vi "PXI-Set AO Gains.vi"(8 "error in (no error)":errorcluster, 11 "AO Tasks":T1[](array[typedef])) -> (0 "error out":errorcluster, 3 "AO Tasks out":T1[](array[typedef]))   [LabVIEW 2020]
uses:
  Type Defs/Task Struct.ctl
  PXI Globals.vi
  <resource>/objmgr/daqmx.rc
panel:
  out "Channels":i32[](array[numeric])
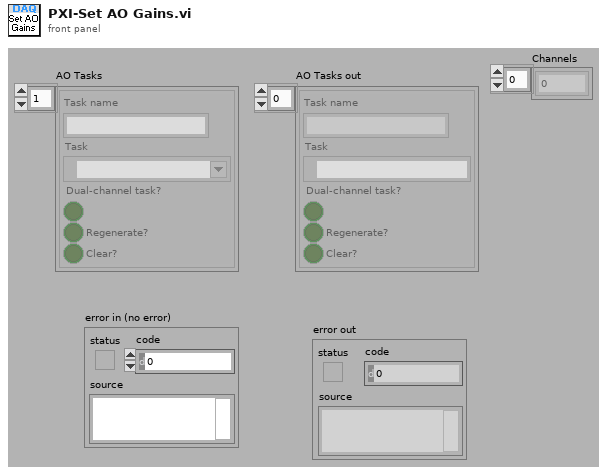
[diagram p1: front panel]
types:
  T1 = typedef "Task Struct.ctl" = cluster{"Task name":string, "Task":refnum<k21>, "Dual-channel task?":bool, "Regenerate?":bool, "Clear?":bool}
  T2 = enum16{"Init", "Write", "Read", "Latch setup", "Compute comp.", "Read 1 Channel"}
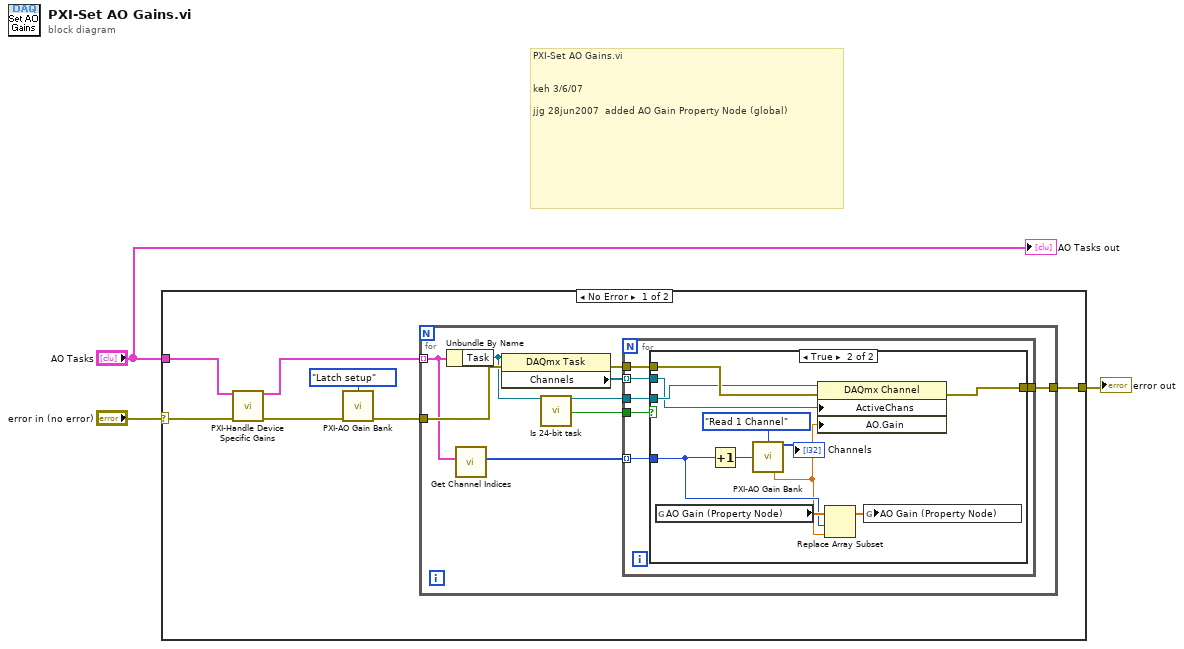
[diagram p0: block diagram]
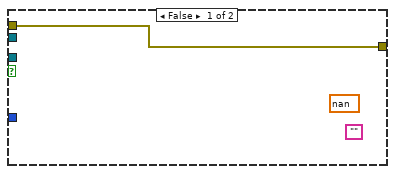
[diagram p2: hidden frame]
diagram:
  # "PXI-Set AO Gains.vi\n\n\nkeh 3/6/07\n\njjg 28jun2007  added AO Gain Property Node (global)"
  n1 = case shown="No Error" "error in (no error)" {
    selector: "error in (no error)" -> [w7 w38]
    tunnel: [w10 w38] -> w2
    tunnel: "AO Tasks" -> [w5 _]
    frame No Error {
      n2 = call "PXI-Handle Device Specific Gains.vi"("AO Tasks in"=w5, "error in (no error)"=w7) -> ("AO Tasks out"=w4:T1[], "error out"=w6:errorcluster)  [unwired: 12 in]
      n3 = call "PXI-AO Gain Bank.vi"("Action"=T2."Latch setup", "error in (no error)"=w6) -> ("error out"=w8:errorcluster)  [unwired: 8 in, 5 out]
      n4 = for {
        tunnel: w4 -> [w15] mode=indexing
        tunnel: w8 -> [w19]
        tunnel: [w16] -> w10
        n5 = Unbundle By Name(w15) -> ("Task"=w12:refnum<k21>)
        n6 = call "Get Channel Indices.vi"("Task Structure"=w15) -> ("Channel Indices"=w14:i32[])  [unwired: 10 in]
        n7 = property class="DAQmx Task"(reference=w12, error in=w19) -> (error out=w18:errorcluster, "Channels"=w17:refnum<k21>[])  [unwired: 1 out]
        n8 = call "Is 24-bit task.vi"("task"=w12) -> ("task out"=w11:refnum<k21>, "is 24bit?"=w13:bool)  [unwired: 9 in, 4 out]
        n9 = for {
          tunnel: w13 -> [w25]
          tunnel: w18 -> [w24]
          tunnel: w17 -> [w23] mode=indexing
          tunnel: [w22] -> w16
          tunnel: w11 -> [w21]
          tunnel: w14 -> [w20] mode=indexing
          n10 = case shown="True" w25 {
            tunnel: w24 -> [w26 w37]
            tunnel: w23 -> [_ w32]
            tunnel: [w26 w36] -> w22
            tunnel: w21 -> [_ w35]
            tunnel: w20 -> [_ w30]
            frame False {
              (unwired) nan ("Numeric")
              (unwired) ""
            }
            frame True {
              n11 = global read "PXI Globals.vi" "AO Gain (Property Node)"() -> (w33:dbl[])
              n12 = Increment(x=w30) -> (x+1=w29:i32)
              n13 = call "PXI-AO Gain Bank.vi"("Action"=T2."Read 1 Channel", "AO channel"=w29) -> ("Channels"=→"Channels":i32[], "Gain 1 channel"=w28:dbl)  [unwired: 8 in, 4 out]
              n14 = property class="DAQmx Channel"(reference=w35, error in=w37, "ActiveChans"=w32, "AO.Gain"=w28) -> (error out=w36:errorcluster)  [unwired: 1 out]
              n15 = Replace Array Subset(array=w33, new element=w28, index=w30) -> (w34:dbl[])
              n16 = global write "PXI Globals.vi" "AO Gain (Property Node)"(w34) -> ()
            }
          }
        }
      }
    }
    frame Error {
    }
  }
  "error out" <- w2
  "AO Tasks out" <- "AO Tasks"
